vi "Example 9 - Case Structures.vi"() -> ()   [LabVIEW 2015]
uses:
  library/Scripting.lvlib
panel:
  in  "Demontrate Default if Unwired?":bool=TRUE
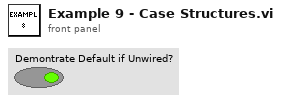
[diagram p1: front panel]
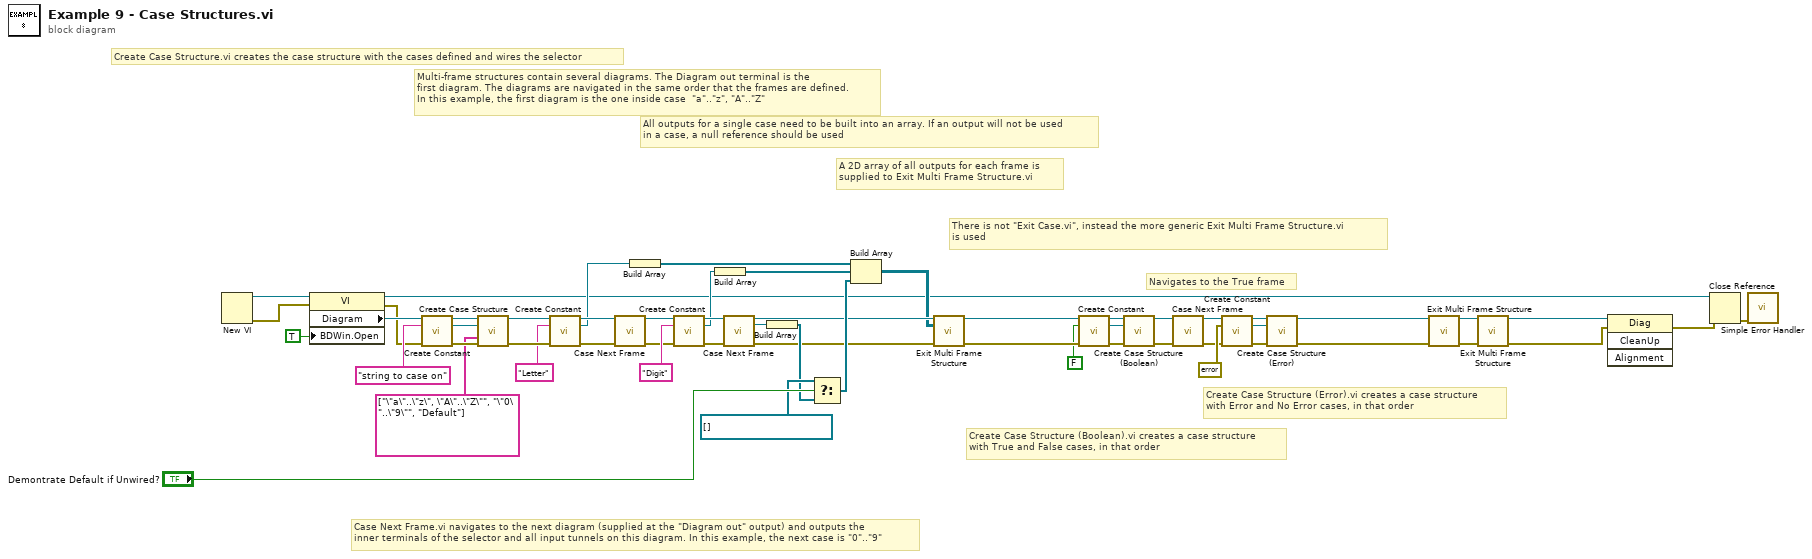
[diagram p0: block diagram]
diagram:
  # "Navigates to the True frame"
  # "Create Case Structure (Error).vi creates a case structure\nwith Error and No Error cases, in that order"
  # "Create Case Structure (Boolean).vi creates a case structure\nwith True and False cases, in that order"
  # "There is not \"Exit Case.vi\", instead the more generic Exit Multi Frame Structure.vi\nis used"
  # "A 2D array of all outputs for each frame is\nsupplied to Exit Multi Frame Structure.vi"
  # "All outputs for a single case need to be built into an array. If an output will not be used\nin a case, a null reference should be used"
  # "Case Next Frame.vi navigates to the next diagram (supplied at the \"Diagram out\" output) and outputs the\ninner terminals of the selector and all input tunnels on this diagram. In this example, the next case is \"0\"..\"9\""
  # "Multi-frame structures contain several diagrams. The Diagram out terminal is the\nfirst diagram. The diagrams are navigated in the same order that the frames are defined.\nIn this example, the first diagram is the one inside case  \"a\"..\"z\", \"A\"..\"Z\""
  # "Create Case Structure.vi creates the case structure with the cases defined and wires the selector"
  n1 = New VI() -> (0:w51:errorcluster, 3:w52:refnum<vi>)  [unwired: 7 in]
  n2 = property class="VI"(reference=w52, error in=w51, "BDWin.Open"=TRUE ("Block Diagram Window:Open")) -> (reference out=w20:refnum<vi>, error out=w48:errorcluster, "Diagram"=w49:refnum<vi>)
  n3 = call "Create Constant.vi"("Diagram in"=w49, "Type"="string to case on", "error in (no error)"=w48) -> ("Diagram out"=w47:refnum<vi>, "Terminal"=w45:refnum<vi>, "error out"=w46:errorcluster)  [unwired: 10 in]
  n4 = call "Create Case Structure.vi"("Diagram in"=w47, "Selector"=w45, "Frames"=string[] ["\"a\"..\"z\", \"A\"..\"Z\"", "\"0\"..\"9\"", "Default"], "error in (no error)"=w46) -> ("Selected Diagram"=w43:refnum<vi>, "error out"=w42:errorcluster)  [unwired: 8 in, 2 out]
  n5 = call "Create Constant.vi"("Diagram in"=w43, "Type"="Letter", "error in (no error)"=w42) -> ("Diagram out"=w41:refnum<vi>, "Terminal"=w33:refnum<vi>, "error out"=w40:errorcluster)  [unwired: 10 in]
  n6 = call "Case Next Frame.vi"("Diagram in"=w41, "error in (no error)"=w40) -> ("Selected Diagram"=w37:refnum<vi>, "error out"=w36:errorcluster)  [unwired: 10 in, 2 out]
  n7 = Build Array(w33) -> (w27:refnum<vi>[])
  n8 = call "Create Constant.vi"("Diagram in"=w37, "Type"="Digit", "error in (no error)"=w36) -> ("Diagram out"=w35:refnum<vi>, "Terminal"=w32:refnum<vi>, "error out"=w34:errorcluster)  [unwired: 10 in]
  n9 = Build Array(w32) -> (w26:refnum<vi>[])
  n10 = call "Case Next Frame.vi"("Diagram in"=w35, "error in (no error)"=w34) -> ("Selected Diagram"=w24:refnum<vi>, "Selector"=w31:refnum<vi>, "error out"=w23:errorcluster)  [unwired: 10 in, 1 out]
  n11 = Build Array(w31) -> (w28:refnum<vi>[])
  n12 = Select(t=refnum<vi>[] [] ("f"), s="Demontrate Default if Unwired?", f=w28) -> (s? t:f=w25:refnum<vi>[])
  n13 = Build Array(w27, w26, w25) -> (w22:refnum<vi>[][])
  n14 = call "Exit Multi Frame Structure.vi"("Diagram in"=w24, "Outputs"=w22, "error in (no error)"=w23) -> ("Diagram out"=w18:refnum<vi>, "error out"=w21:errorcluster)  [unwired: 10 in, 1 out]
  n15 = call "Create Constant.vi"("Diagram in"=w18, "Type"=FALSE, "error in (no error)"=w21) -> ("Diagram out"=w15:refnum<vi>, "Terminal"=w14:refnum<vi>, "error out"=w19:errorcluster)  [unwired: 10 in]
  n16 = call "Create Case Structure (Boolean).vi"("Diagram in"=w15, "Selector"=w14, "error in (no error)"=w19) -> ("Selected Diagram"=w2:refnum<vi>, "error out"=w16:errorcluster)  [unwired: 9 in, 2 out]
  n17 = call "Case Next Frame.vi"("Diagram in"=w2, "error in (no error)"=w16) -> ("Selected Diagram"=w1:refnum<vi>, "error out"=w3:errorcluster)  [unwired: 10 in, 2 out]
  n18 = call "Create Constant.vi"("Diagram in"=w1, "Type"=errorcluster {"status"=FALSE, "code"=0, "source"=""} ("error constant"), "error in (no error)"=w3) -> ("Diagram out"=w11:refnum<vi>, "Terminal"=w10:refnum<vi>, "error out"=w13:errorcluster)  [unwired: 10 in]
  n19 = call "Create Case Structure (Error).vi"("Diagram in"=w11, "Selector"=w10, "error in (no error)"=w13) -> ("Selected Diagram"=w7:refnum<vi>, "error out"=w12:errorcluster)  [unwired: 9 in, 2 out]
  n20 = call "Exit Multi Frame Structure.vi"("Diagram in"=w7, "error in (no error)"=w12) -> ("Diagram out"=w5:refnum<vi>, "error out"=w8:errorcluster)  [unwired: 11 in, 1 out]
  n21 = call "Exit Multi Frame Structure.vi"("Diagram in"=w5, "error in (no error)"=w8) -> ("Diagram out"=w4:refnum<vi>, "error out"=w6:errorcluster)  [unwired: 11 in, 1 out]
  n22 = invoke class="Diag" method="CleanUp"(reference=w4, error in=w6) -> (error out=w53:errorcluster)  [unwired: 2 in, 3 out]
  n23 = Close Reference(reference=w20, error in (no error)=w53) -> (error out=w54:errorcluster)
  n24 = call <vilib>:"Simple Error Handler.vi"("error in (no error)"=w54) -> ()  [unwired: 4 in, 5 out]
